vi "BrokerConnect.vi"(0 "mqtt in":refnum<class "MQTT Client.lvclass">, 11 "error in (no error)":errorcluster) -> (4 "mqtt out":refnum<class "MQTT Client.lvclass">, 15 "error out":errorcluster)   [LabVIEW 2020, in "MQTT Client.lvclass"]
uses:
  MQTT Client.lvclass
  MQTT Client.lvclass/MQTT Client.ctl
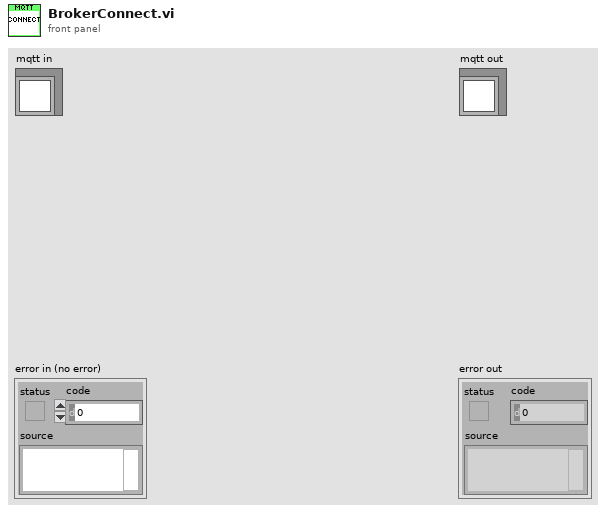
[diagram p1: front panel]
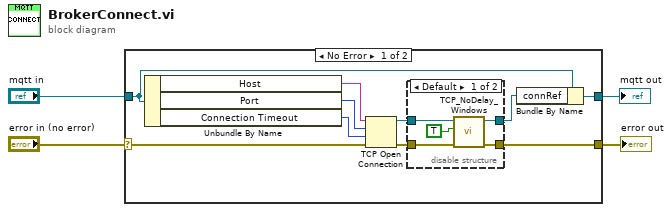
[diagram p0: block diagram]
diagram:
  n1 = case shown="No Error" "error in (no error)" {
    selector: "error in (no error)" -> [w9 w23]
    tunnel: [w12 w23] -> w3
    tunnel: [w10 w22] -> w1
    tunnel: "mqtt in" -> [w8 w22]
    frame No Error {
      n2 = Unbundle By Name(w8) -> ("Host"=w7:string, "Port"=w6:u16, "Connection Timeout"=w5:i32)
      n3 = TCP Open Connection(address=w7, remote port or service name=w6, timeout ms (60000)=w5, error in (no error)=w9) -> (connection ID=w14:refnum<k5>, error out=w13:errorcluster)  [unwired: 1 in]
      n4 = disable-structure shown="Default" {
        disable-tunnel: w14 -> [w19 w21]
        disable-tunnel: w13 -> [w18 w20]
        disable-tunnel: [w17 w20] -> w12
        disable-tunnel: [w15 w21] -> w11
        frame condition #0 (active) {
          n5 = call "TCP_NoDelay_Windows.vi"("error in (no error)"=w18, "TCP_NODELAY (true)"=TRUE, "connID"=w19) -> ("error out"=w17:errorcluster, "connID 2"=w15:refnum<k5>)  [unwired: 3 in]
        }
        frame condition #1 {
        }
      }
      n6 = Bundle By Name(cluster=w8, "connRef"=w11) -> (w10:refnum<class "MQTT Client.lvclass">)
    }
    frame Error {
    }
  }
  "error out" <- w3
  "mqtt out" <- w1
